vi "外观 2.vi"(0 "Data In":T4 caption="数据输入" {"测量数据区"."单位" items=["ug/L", "mg/L", "ppm", "mg/m3", "cm", "ppb", "ug/m3", "%", "nmol/mol", "umol/mol", "MPN/L", "MPN/100ml", "ng/m3", "NTU", "无量纲", "ms/cm", "us/cm", "℃", "mV", "万个/L"]}, 2 "Display State In":T2 caption="显示状态输入", 3 "Container State":T3 caption="容器状态") -> (6 "Data Out":T4 caption="数据输出" {"测量数据区"."单位" items=["ug/L", "mg/L", "ppm", "mg/m3", "cm", "ppb", "ug/m3", "%", "nmol/mol", "umol/mol", "MPN/L", "MPN/100ml", "ng/m3", "NTU", "无量纲", "ms/cm", "us/cm", "℃", "mV", "万个/L"]}, 7 "Display State Out":T2 caption="显示状态输出", 8 "Action":T1 caption="动作")   [LabVIEW 2016, in "总磷氨氮测量数据.xctl"]
uses:
  <vilib>/_xctls/Container State.ctl
  <vilib>/_xctls/Action.ctl
  <vilib>/_xctls/XControlSupport.lvlib
panel:
  out "数据标识":string
  out "实测值":string
  out "数据时间":string
  out "单位":string
  out "因子编码":string
  # "因子编码:"
  # "单位:"
  # "数据时间:"
  # "实测值:"
  # "数据标识:"
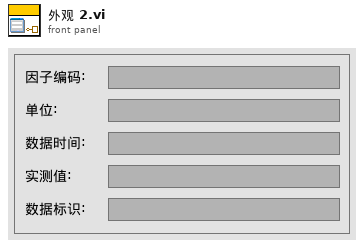
[diagram p1: front panel]
types:
  T1 = typedef "XControlSupport.lvlib/Action.ctl" = cluster{"Data Changed?":bool, "State Changed?":bool, "Action Name":string}
  T2 = typedef "总磷氨氮测量数据.xctl/状态 1.ctl" = cluster{"Numeric":dbl}
  T3 = typedef "XControlSupport.lvlib/Container State.ctl" = cluster{"Indicator?":bool, "Run Mode?":bool, " Refnum":refnum<vi>}
  T4 = typedef "总磷氨氮测量数据.xctl/数据 1.ctl" = cluster{"flowid":u16, "测量精度":u16, "测量数据区":cluster{"因子编码":u32, "单位":u16, "标样参考值":sgl, "水样数据时间":timestamp, "水样实测值":sgl, "水样数据标识":string, "标样数据时间":timestamp, "标样实测值":sgl, "标样数据标识":string, "空白数据时间":timestamp, "空白实测值":sgl, "空白数据标识":string, "零点核查数据时间":timestamp, "零点核查实测值":sgl, "零点核查数据标识":string, "跨度核查数据时间":timestamp, "跨度核查实测值":sgl, "跨度核查数据标识":string, "加标回收数据时间":timestamp, "加标回收实测值":sgl, "加标回收数据标识":string, "平行样数据时间":timestamp, "平行样实测值":sgl, "平行样数据标识":string, "F0":sgl, "F1":sgl, "F2":sgl, "F3":sgl, "F4":sgl, "F5":sgl, "F6":sgl, "F7":sgl, "温度":sgl, "湿度":sgl, "X值":sgl}}
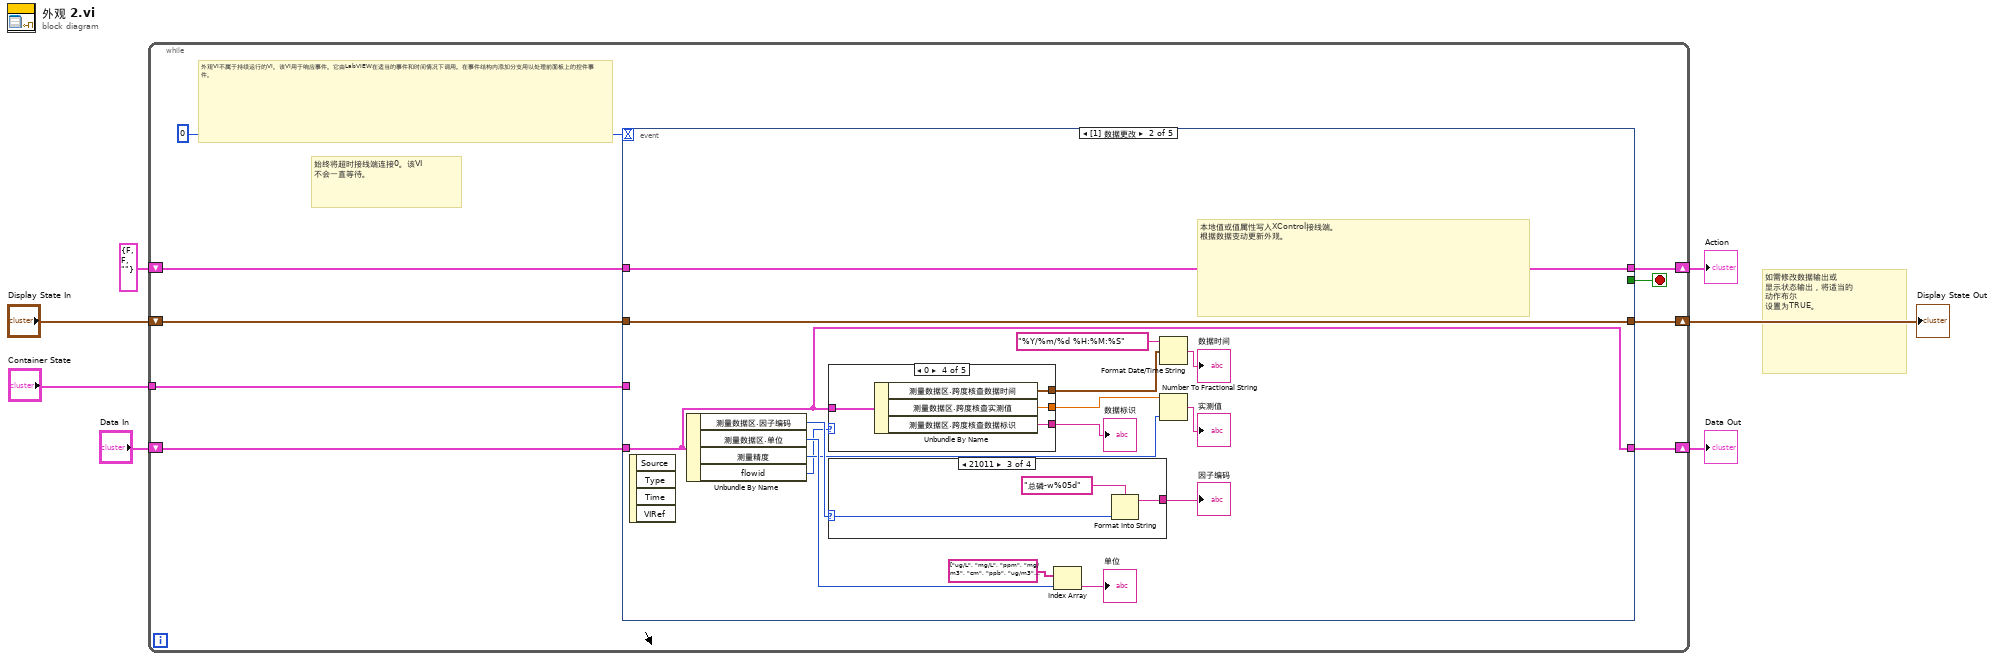
[diagram p0: block diagram]
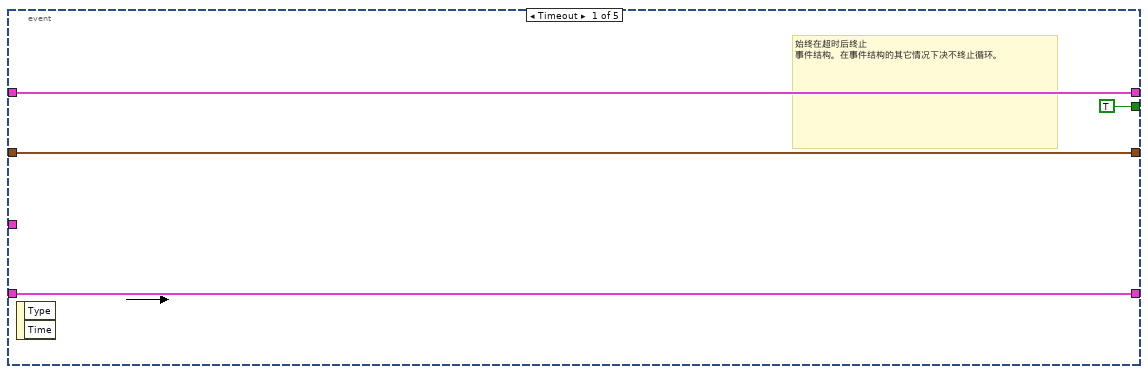
[diagram p2: hidden frame]
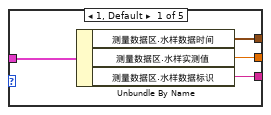
[diagram p3: hidden frame]
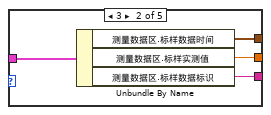
[diagram p4: hidden frame]
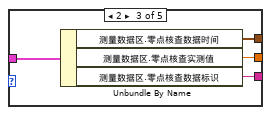
[diagram p5: hidden frame]
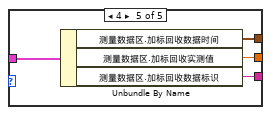
[diagram p6: hidden frame]
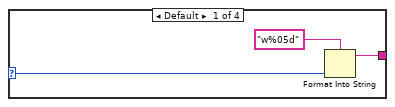
[diagram p7: hidden frame]
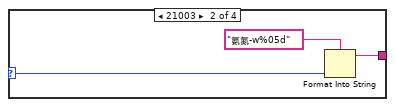
[diagram p8: hidden frame]
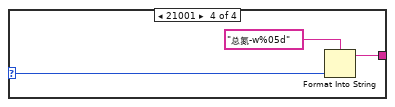
[diagram p9: hidden frame]
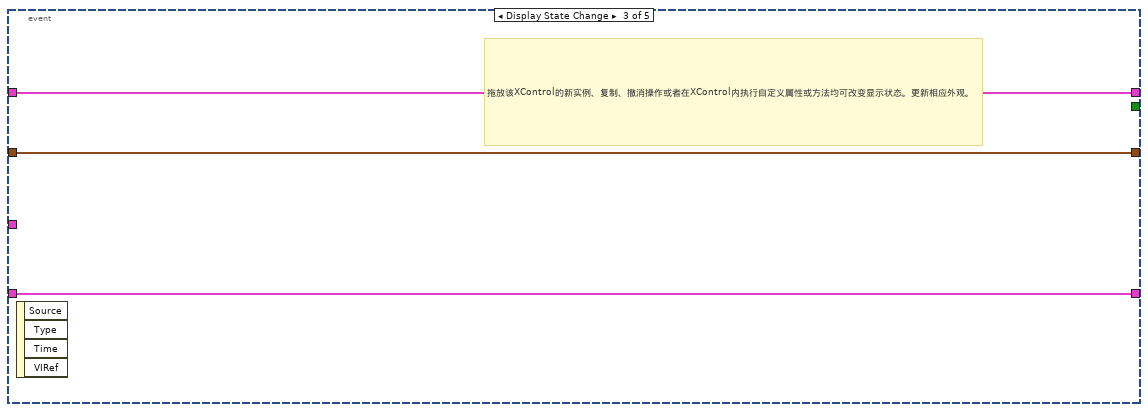
[diagram p10: hidden frame]
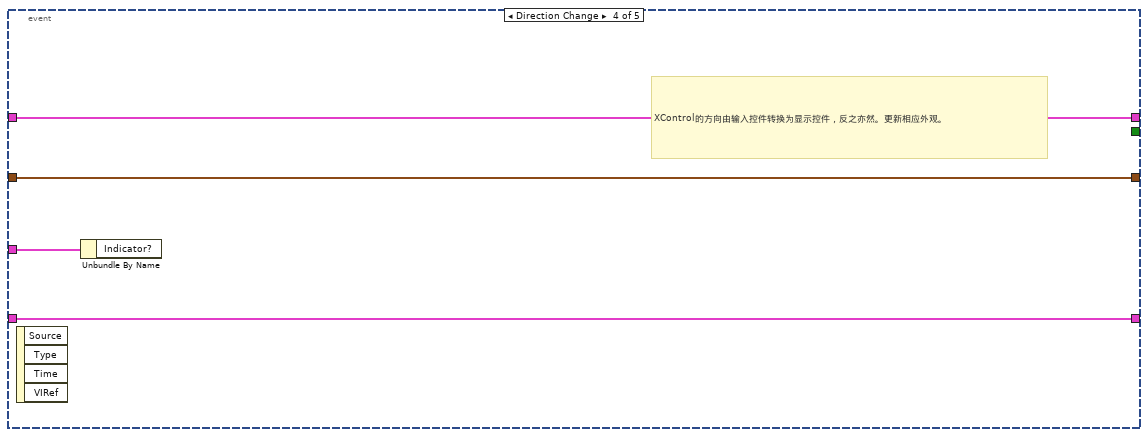
[diagram p11: hidden frame]
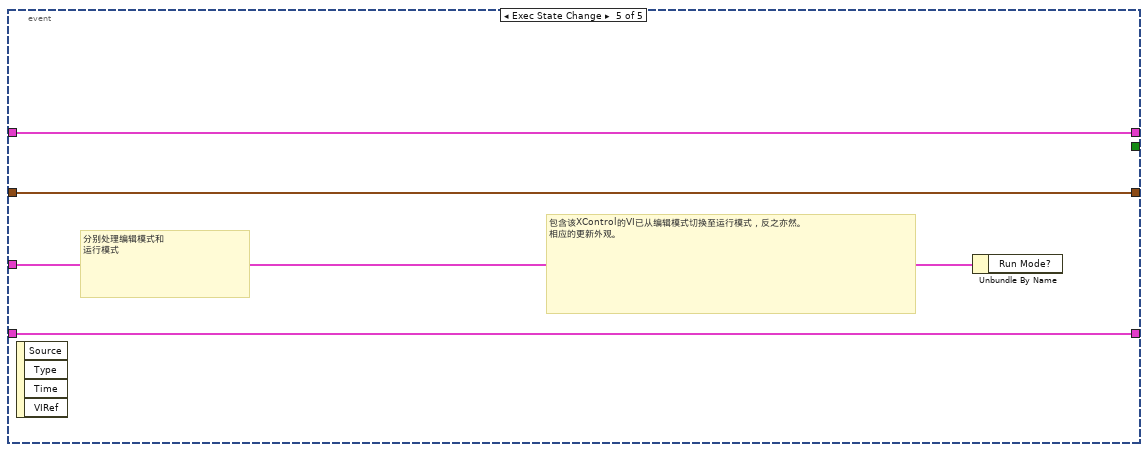
[diagram p12: hidden frame]
diagram:
  # "如需修改数据输出或\n显示状态输出，将适当的\n动作布尔\n设置为TRUE。"
  n1 = while {
    shift-right: [w15] -> w4
    shift-left: "Display State In" -> [w16]
    tunnel: "Container State" -> [w12]
    shift-right: [w10] -> w7
    shift-left: "Data In" -> [w11]
    shift-right: [w8] -> w2
    shift-left: T1 {"Data Changed?"=FALSE, "State Changed?"=FALSE, "Action Name"=""} ("Action") -> [w9]
    stop <- w14 stop-if-true
    # "外观VI不属于持续运行的VI。该VI用于响应事件。它由LabVIEW在适当的事件和时间情况下调用。在事件结构内添加分支用以处理前面板上的控件事件。"
    # "始终将超时接线端连接0。该VI\n不会一直等待。"
    n2 = event shown="[1] 数据更改" {
      selector: _ -> [_ _ _ _ _]
      dyn-events: _ -> [_ _ _ _ _]
      timeout: 0 -> [_ _ _ _ _]
      tunnel: w16 -> [w18 w36 w71 w74 w78]
      tunnel: [w18 w36 w71 w74 w78] -> w15
      tunnel: [TRUE _ _ _ _] -> w14
      tunnel: w12 -> [_ _ _ w75 w79]
      tunnel: w11 -> [w17 w25 w70 w73 w77]
      tunnel: [w17 w25 w70 w73 w77] -> w10
      tunnel: [w19 w35 w69 w72 w76] -> w8
      tunnel: w9 -> [w19 w35 w69 w72 w76]
      event Timeout {
        # "始终在超时后终止\n事件结构。在事件结构的其它情况下决不终止循环。"
        n3 = event-data() -> ()  [unwired: 1 in, 2 out]
      }
      event Data Change {
        # "本地值或值属性写入XControl接线端。\n根据数据变动更新外观。"
        n4 = event-data() -> ()  [unwired: 1 in, 4 out]
        n5 = Unbundle By Name(w25) -> ("测量数据区.因子编码"=w31:u32, "测量数据区.单位"=w28:u16, "测量精度"=w26:u16, "flowid"=w21:u16)
        n6 = case shown="0" w21 {
          tunnel: w25 -> [w40 w44 w48 w52 w56]
          tunnel: [w39 w43 w47 w51 w55] -> w24
          tunnel: [w38 w42 w46 w50 w53] -> w22
          tunnel: [w37 w41 w45 w49 w54] -> w23
          frame 1, Default {
            n7 = Unbundle By Name(w40) -> ("测量数据区.水样数据时间"=w39:timestamp, "测量数据区.水样实测值"=w38:sgl, "测量数据区.水样数据标识"=w37:string)
          }
          frame 3 {
            n8 = Unbundle By Name(w44) -> ("测量数据区.标样数据时间"=w43:timestamp, "测量数据区.标样实测值"=w42:sgl, "测量数据区.标样数据标识"=w41:string)
          }
          frame 2 {
            n9 = Unbundle By Name(w48) -> ("测量数据区.零点核查数据时间"=w47:timestamp, "测量数据区.零点核查实测值"=w46:sgl, "测量数据区.零点核查数据标识"=w45:string)
          }
          frame 0 {
            n10 = Unbundle By Name(w52) -> ("测量数据区.跨度核查数据时间"=w51:timestamp, "测量数据区.跨度核查实测值"=w50:sgl, "测量数据区.跨度核查数据标识"=w49:string)
          }
          frame 4 {
            n11 = Unbundle By Name(w56) -> ("测量数据区.加标回收数据时间"=w55:timestamp, "测量数据区.加标回收实测值"=w53:sgl, "测量数据区.加标回收数据标识"=w54:string)
          }
        }
        "数据标识" <- w23
        n12 = case shown="21011" w31 {
          selector: w31 -> [w58 w61 w64 w67]
          tunnel: [w57 w60 w63 w66] -> w30
          frame Default {
            n13 = Format Into String(format string="w%05d" ("格式字符串"), w58) -> (resulting string=w57:string)  [unwired: 2 in, 1 out]
          }
          frame 21003 {
            n14 = Format Into String(format string="氨氮-w%05d" ("格式字符串"), w61) -> (resulting string=w60:string)  [unwired: 2 in, 1 out]
          }
          frame 21011 {
            n15 = Format Into String(format string="总磷-w%05d" ("格式字符串"), w64) -> (resulting string=w63:string)  [unwired: 2 in, 1 out]
          }
          frame 21001 {
            n16 = Format Into String(format string="总氮-w%05d" ("格式字符串"), w67) -> (resulting string=w66:string)  [unwired: 2 in, 1 out]
          }
        }
        "因子编码" <- w30
        n17 = Index Array(array=string[] ["ug/L", "mg/L", "ppm", "mg/m3", "cm", "ppb", "ug/m3", "%", "nmol/mol", "umol/mol", "MPN/L", "MPN/100ml", "ng/m3", "NTU", "无量纲", "ms/cm", "us/cm", "℃", "mV", "万个/L"] ("字符串[]"), index=w28) -> (element=→"单位":string)
        n18 = Format Date/Time String(time format string (%c)="%Y/%m/%d %H:%M:%S" ("时间格式字符串(%c)"), seconds (now)=w24) -> (date/time string=→"数据时间":string)  [unwired: 1 in]
        n19 = Number To Fractional String(number=w22, precision (6)=w26) -> (F-format string=→"实测值":string)  [unwired: 2 in]
      }
      event Display State Change {
        # "拖放该XControl的新实例、复制、撤消操作或者在XControl内执行自定义属性或方法均可改变显示状态。更新相应外观。"
        n20 = event-data() -> ()  [unwired: 1 in, 4 out]
      }
      event Direction Change {
        # "XControl的方向由输入控件转换为显示控件，反之亦然。更新相应外观。"
        n21 = event-data() -> ()  [unwired: 1 in, 4 out]
        n22 = Unbundle By Name(w75) -> ()  [unwired: 1 out]
      }
      event Exec State Change {
        # "包含该XControl的VI已从编辑模式切换至运行模式，反之亦然。\n相应的更新外观。"
        # "分别处理编辑模式和\n运行模式"
        n23 = event-data() -> ()  [unwired: 1 in, 4 out]
        n24 = Unbundle By Name(w79) -> ()  [unwired: 1 out]
      }
    }
  }
  "Display State Out" <- w4
  "Data Out" <- w7
  "Action" <- w2
